vi "Read ADC.vi"(8 "error in (no error)":errorcluster, 10 "Channel":u8, 11 "Cypress CY8CKIT-059 in":refnum<class "Cypress CY8CKIT-059.lvclass">) -> (0 "error out":errorcluster, 1 "Response":string, 2 "ADC Out":u16, 3 "Cypress CY8CKIT-059 out":refnum<class "Cypress CY8CKIT-059.lvclass">)   [LabVIEW 2020, in "Cypress CY8CKIT-059.lvclass"]
doc: "Sends \"Read ADC\" command to target device, it returns the value of ADC or an error if target response is invalid or it doesn't respond."
uses:
  Cypress CY8CKIT-059.lvclass
  Controls/Device Code.ctl
  Controls/Device Command Code.ctl
  Cypress CY8CKIT-059.lvclass/Cypress CY8CKIT-059.ctl
  ab5203b5-33f3-45f2-a33d-3186aee358c8.vi
  Read Serial Port.vi
  Write Serial Port.vi
  <vilib>/Utility/error.llb/Error Cluster From Error Code.vi
  <vilib>/ErrorRing/Error Ring.xnode
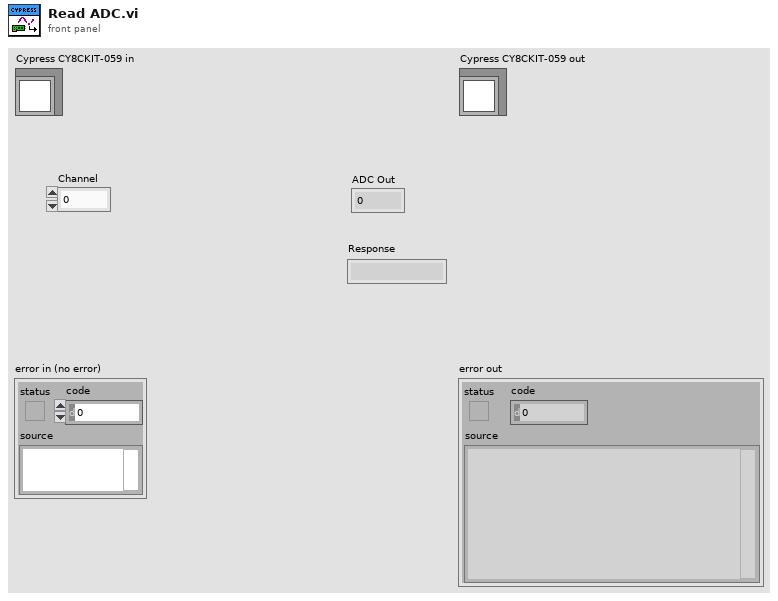
[diagram p1: front panel]
types:
  T1 = typedef "Device Command Code.ctl" = string
  T2 = typedef "Device Code.ctl" = string
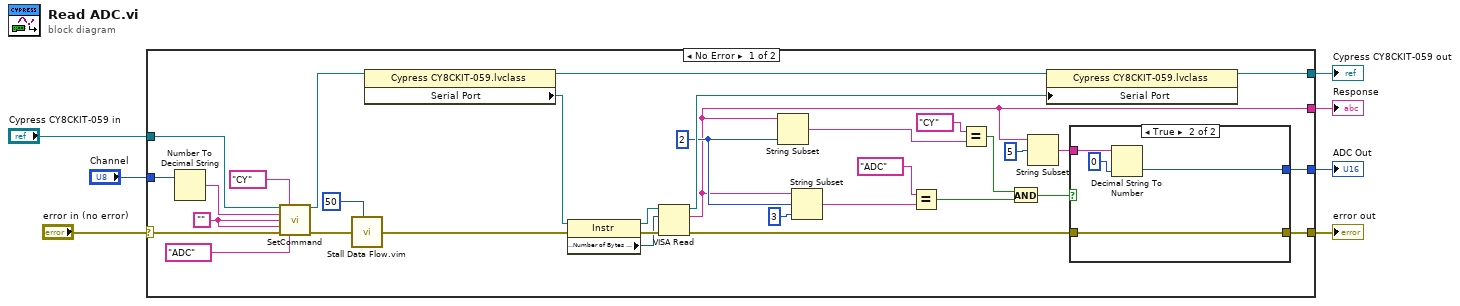
[diagram p0: block diagram]
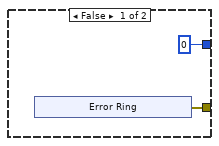
[diagram p2: hidden frame]
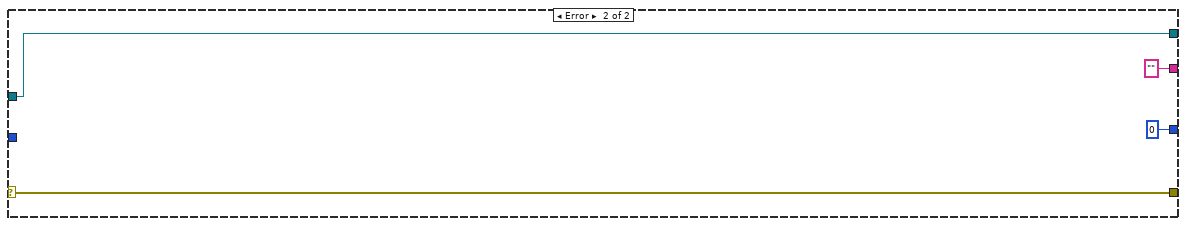
[diagram p3: hidden frame]
diagram:
  n1 = case shown="No Error" "error in (no error)" {
    selector: "error in (no error)" -> [w40 w54]
    tunnel: [w32 w55] -> w6
    tunnel: "Cypress CY8CKIT-059 in" -> [w38 w55]
    tunnel: [w10 w54] -> w4
    tunnel: "Channel" -> [w9 _]
    tunnel: [w21 "" ("read buffer")] -> w2
    tunnel: [w12 u16 0] -> w1
    frame No Error {
      w24 = 2 ("length (rest)")
      w34 = ""
      n2 = Number To Decimal String(number=w9) -> (decimal integer string=w8:string)  [unwired: 1 in]
      n3 = call-dynamic "SetCommand.vi"("Cypress CY8CKIT-059 in"=w38, "Device Code"=T2 "CY", "Parameter 1"=w8, "Parameter 2"=w34, "Parameter 3"=w34, "error in (no error)"=w40, "Command Code"=T1 "ADC") -> ("Cypress CY8CKIT-059 out"=w37:refnum<class "Cypress CY8CKIT-059.lvclass">, "error out"=w39:errorcluster)  [unwired: 6 in, 1 out]
      n4 = call "Stall Data Flow.vim"("value in"=w39, "milliseconds to wait"=u32 50) -> ("value out"=w29:errorcluster)  [unwired: 1 out]
      n5 = property class="Cypress CY8CKIT-059.lvclass"(reference=w37) -> (reference out=w33:refnum<class "Cypress CY8CKIT-059.lvclass">, "Serial Port"=w26:refnum<visa-resource-name>)  [unwired: 1 in, 1 out]
      n6 = property class="Instr"(reference=w26, error in=w29) -> (reference out=w25:refnum<visa-resource-name>, error out=w28:errorcluster, "Serial Settings:Number of Bytes at Serial Port"=w27:u32)
      n7 = VISA Read(VISA resource name=w25, byte count=w27, error in (no error)=w28) -> (VISA resource name out=w30:refnum<visa-resource-name>, read buffer=w21:string, error out=w11:errorcluster)  [unwired: 1 out]
      n8 = String Subset(string=w21, length (rest)=w24) -> (substring=w20:string)  [unwired: 1 in]
      n9 = String Subset(string=w21, offset (0)=w24, length (rest)=3 ("length (rest)")) -> (substring=w18:string)
      n10 = Equal?(x=T1 "ADC" ("Command Code"), y=w18) -> (x = y?=w16:bool)
      n11 = Equal?(x=T2 "CY" ("Device Code"), y=w20) -> (x = y?=w15:bool)
      n12 = And(x=w15, y=w16) -> (x .and. y?=w14:bool)
      n13 = String Subset(string=w21, offset (0)=5) -> (substring=w13:string)  [unwired: 1 in]
      n14 = property class="Cypress CY8CKIT-059.lvclass"(reference=w33, "Serial Port"=w30) -> (reference out=w32:refnum<class "Cypress CY8CKIT-059.lvclass">)  [unwired: 1 in, 1 out]
      n15 = case shown="True" w14 {
        tunnel: w13 -> [_ w51]
        tunnel: [u16 0 w49] -> w12
        tunnel: w11 -> [_ w48]
        tunnel: [w41 w48] -> w10
        frame False {
          n16 = xnode "Error Ring"() -> ("error out"=w41:errorcluster)
        }
        frame True {
          n17 = Decimal String To Number(string=w51, default (0L)=u16 0 ("default (0 I32)")) -> (number=w49:u16)  [unwired: 1 in, 1 out]
        }
      }
    }
    frame Error {
    }
  }
  "error out" <- w4
  "Cypress CY8CKIT-059 out" <- w6
  "Response" <- w2
  "ADC Out" <- w1
